vi "02 Valve Test.vi"() -> ()   [LabVIEW 2012]
uses:
  Agilent Channel Definition.ctl
  Drivers/Agilent 34970/Agilent 34970.lvlib
panel:
  in  "Start Button 1-12":bool[](array[boolean])
  out "Max Valves":bool
  out "Agilent Array":refnum<visa-resource-name>[](array[refnum])
  out "Chan Array":string[](array[string])
  in  "Current Per Valve":dbl=0.42
  in  "Current Limit":dbl=1.0
  out "Channel":string
  in  "Walk Time":u32=20000
  out "Agilent Used":string
  in  "TEST TYPE":bool
  in  "Cycles":i32=10
  in  "OK":bool
  in  "One Shot Time":dbl=2000.0
  in  "Valves 41-50":bool[](array[boolean])
  in  "Valves 51-56":bool[](array[boolean])
  in  "Valves 31-40":bool[](array[boolean])
  in  "Valves 21-30":bool[](array[boolean])
  in  "Valves 11-20":bool[](array[boolean])
  in  "Vavles 1-10":bool[](array[boolean])
  out "error out":errorcluster
  in  "error in (no error)":errorcluster
  out "Station In":string
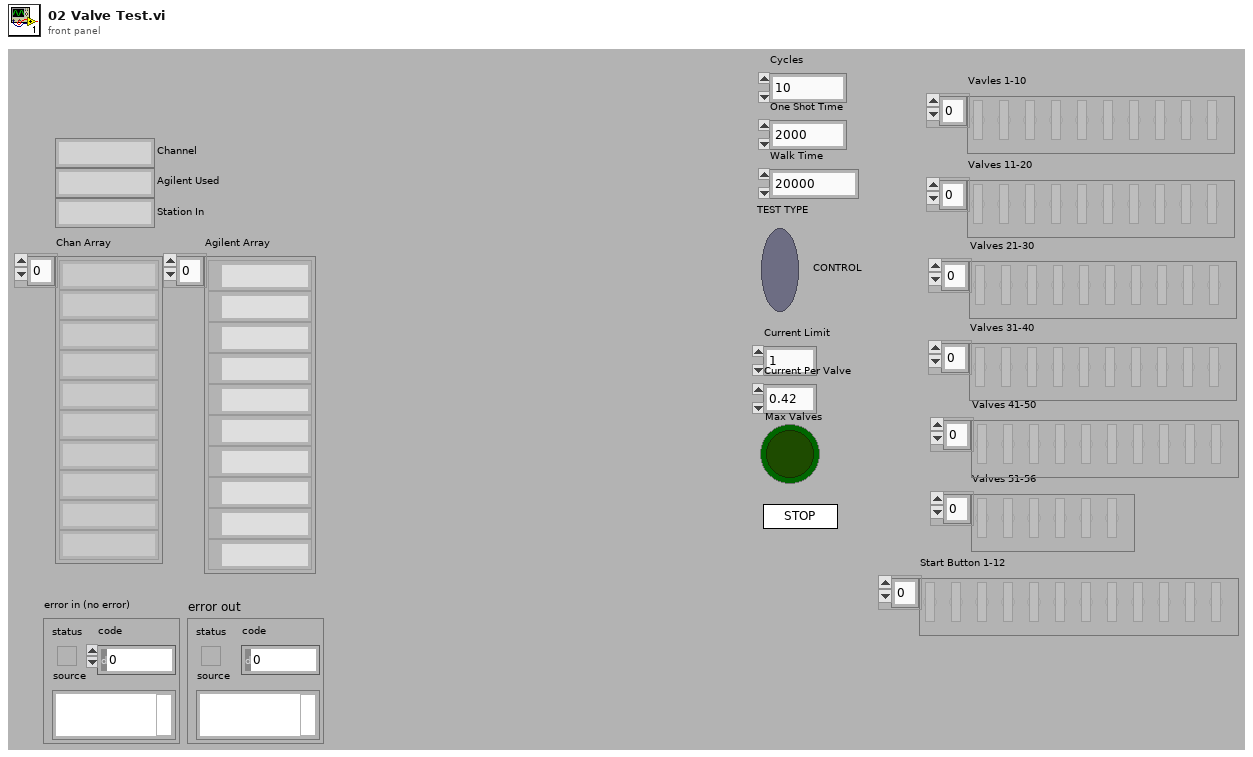
[diagram p1: front panel]
types:
  T1 = typedef "Agilent Channel Definition.ctl" = cluster{"Channel":string, "Station":string, "Label":string, "Agilent Station":string}
  T2 = enum32{"invalid app kind", "Development System", "Run Time System", "Student Edition", "Embedded LabVIEW", "Evaluation", "Custom"}
  T3 = enum32{"Invalid", "Standard", "Closed", "Hidden", "Minimized", "Maximized"}
  T4 = cluster{"Core":cluster{"Current VI Reference":refnum<vi>, "Close Panel on Exit?":bool}, "Valve Array":bool[], "Agilent":refnum<visa-resource-name>, "Channel":string}
  T5 = cluster{"Current VI Reference":refnum<vi>, "Close Panel on Exit?":bool}
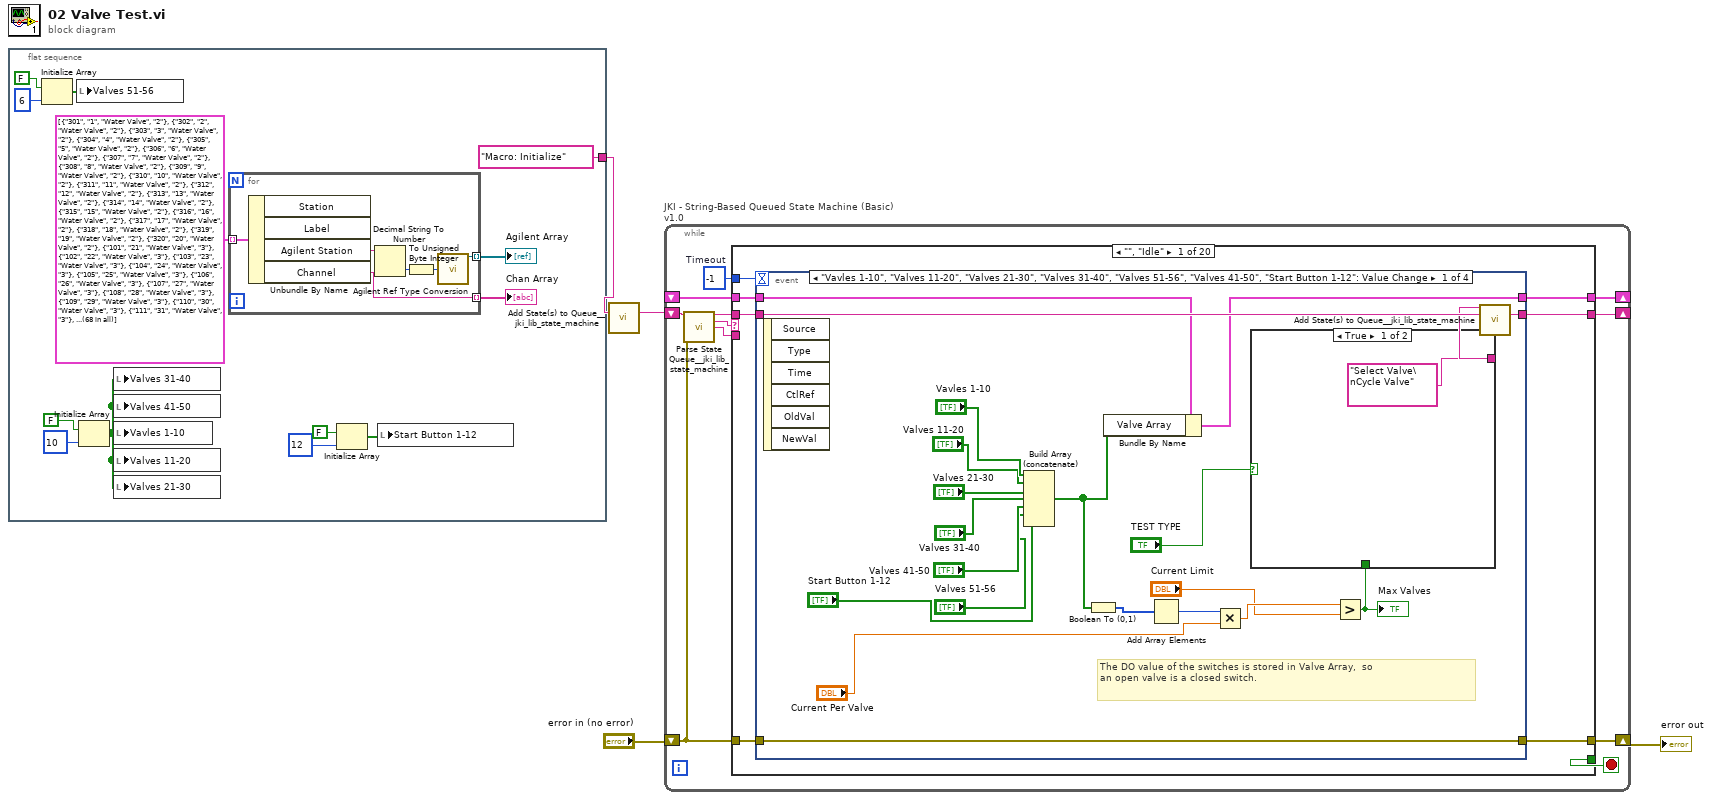
[diagram p0: block diagram]
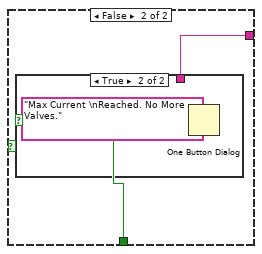
[diagram p2: hidden frame]
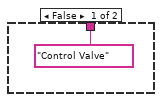
[diagram p3: hidden frame]
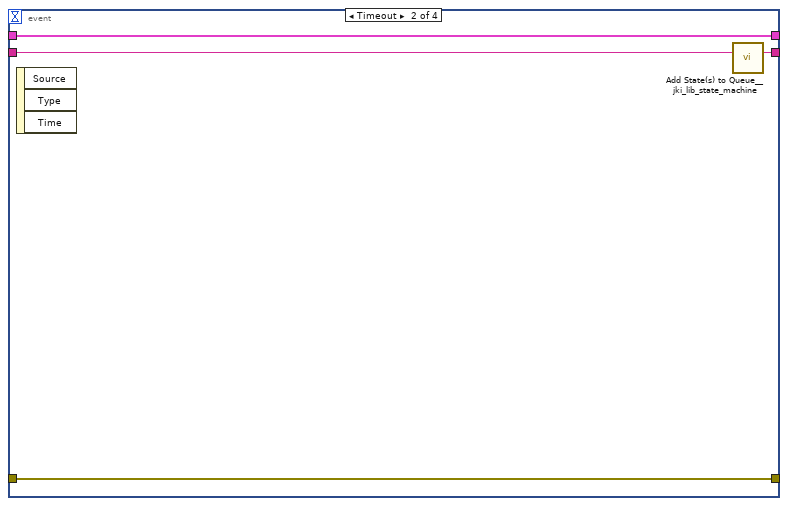
[diagram p4: hidden frame]
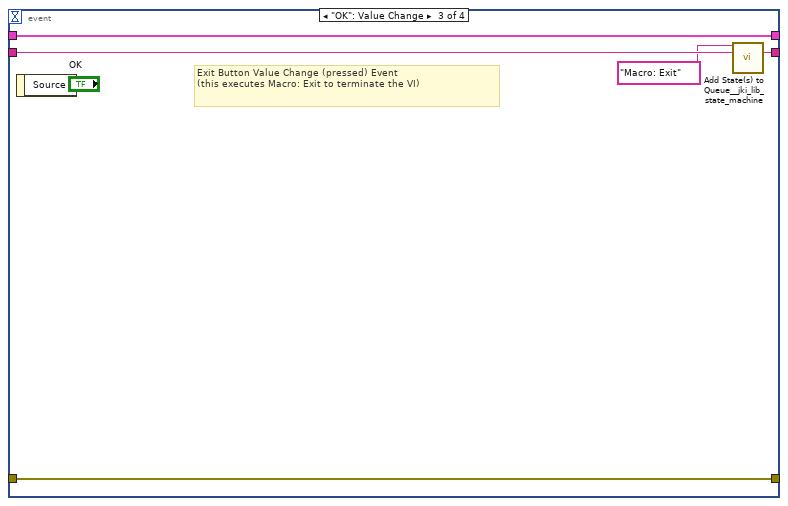
[diagram p5: hidden frame]
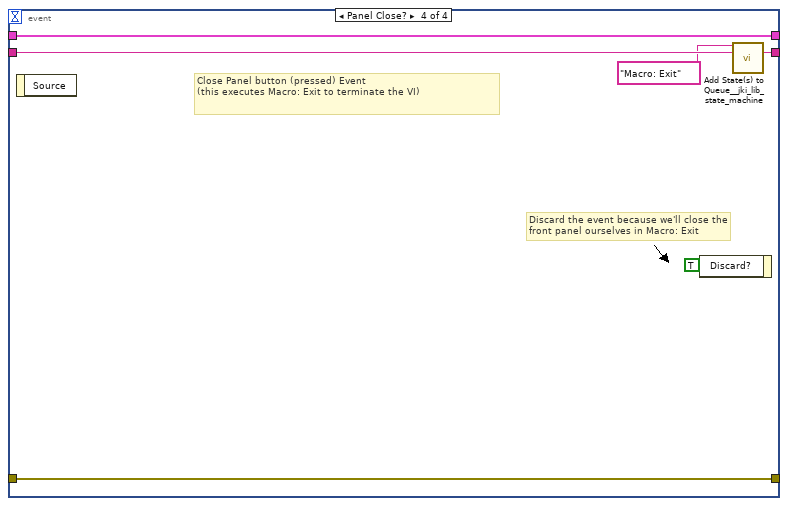
[diagram p6: hidden frame]
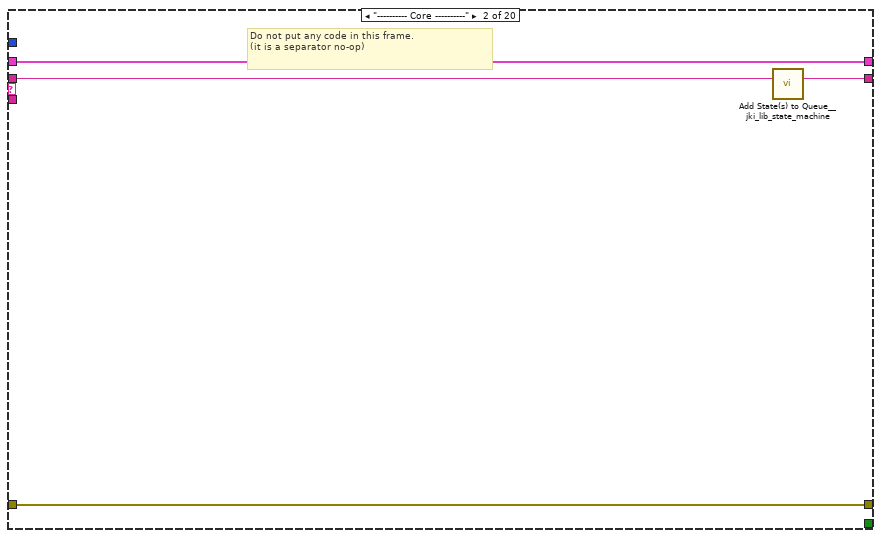
[diagram p7: hidden frame]
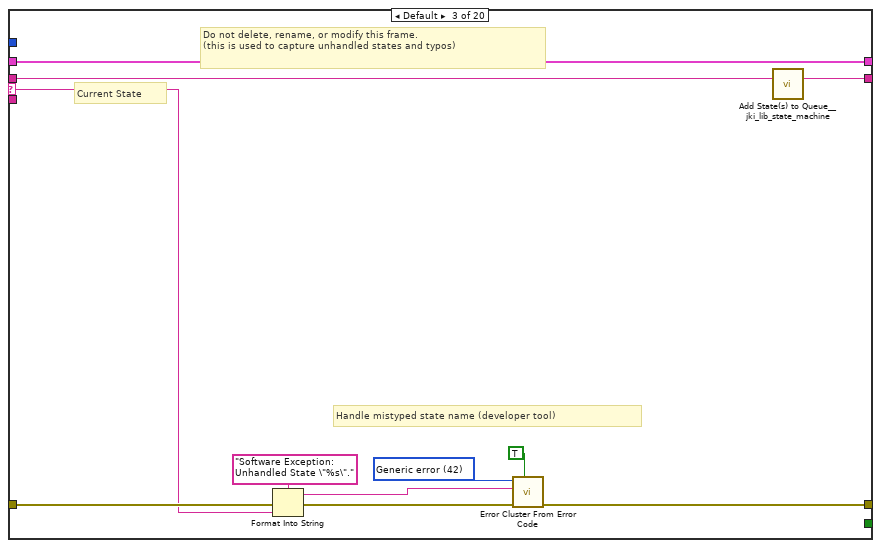
[diagram p8: hidden frame]
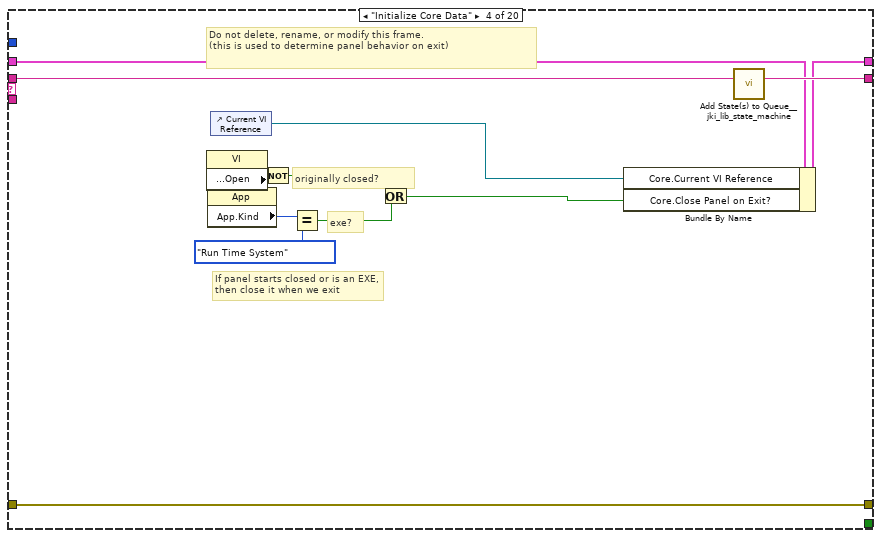
[diagram p9: hidden frame]
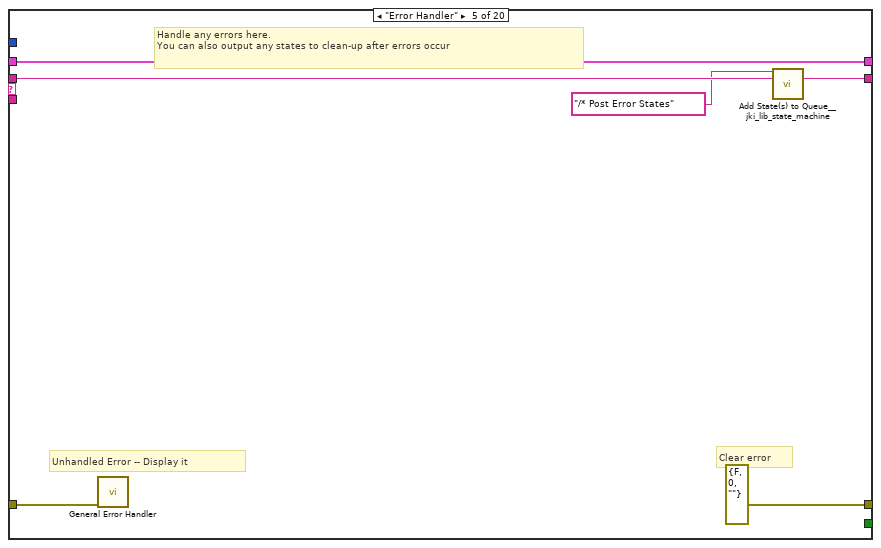
[diagram p10: hidden frame]
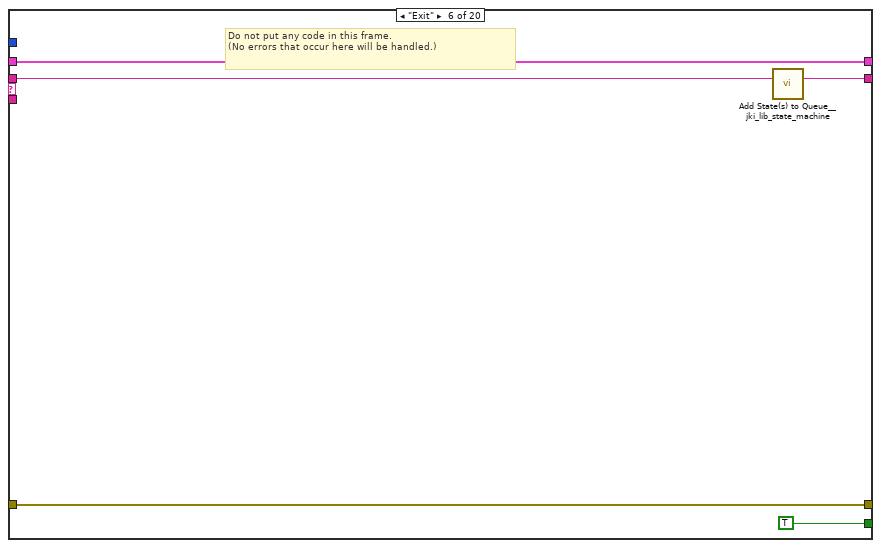
[diagram p11: hidden frame]
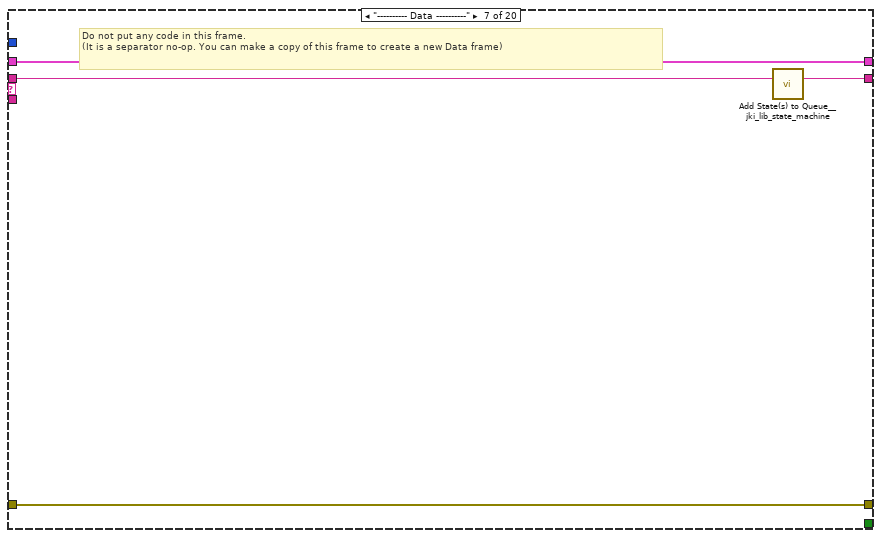
[diagram p12: hidden frame]
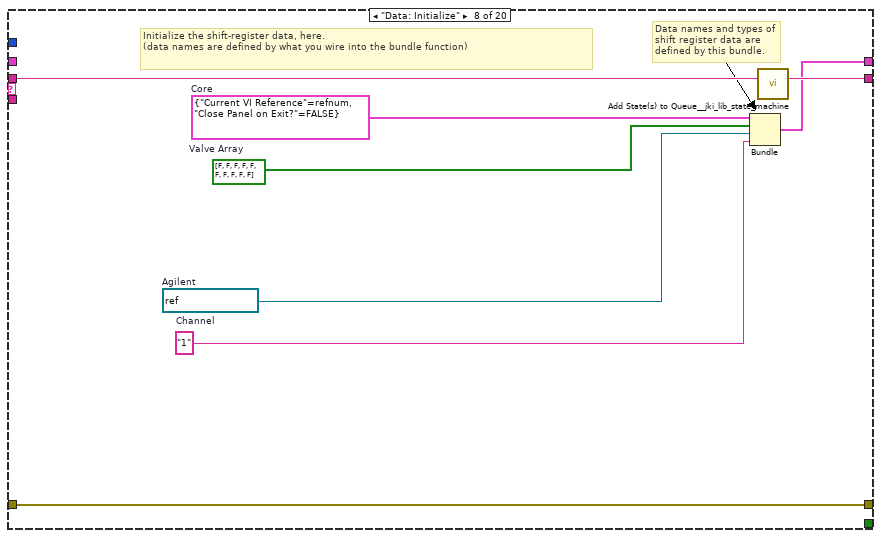
[diagram p13: hidden frame]
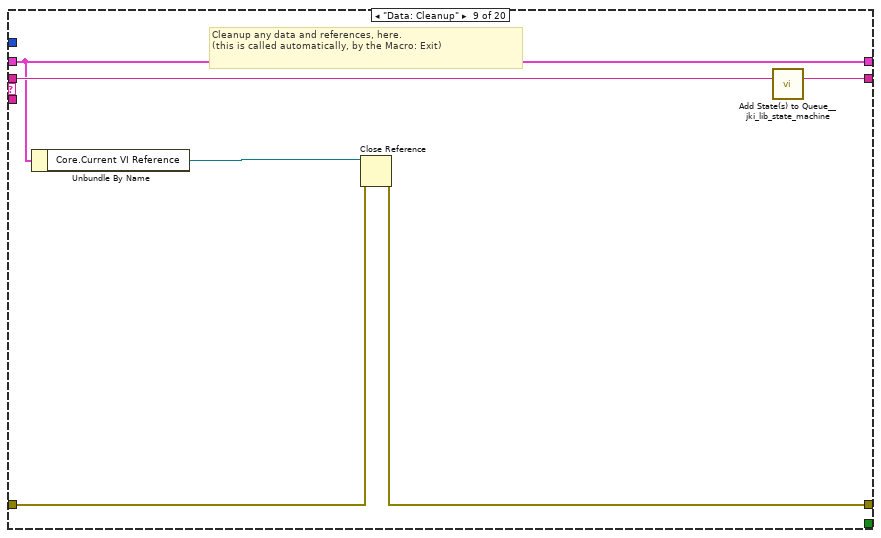
[diagram p14: hidden frame]
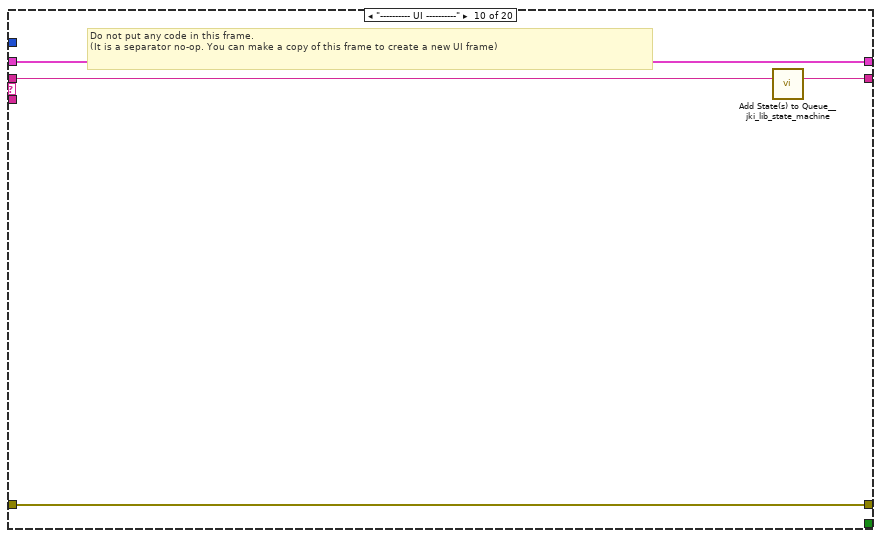
[diagram p15: hidden frame]
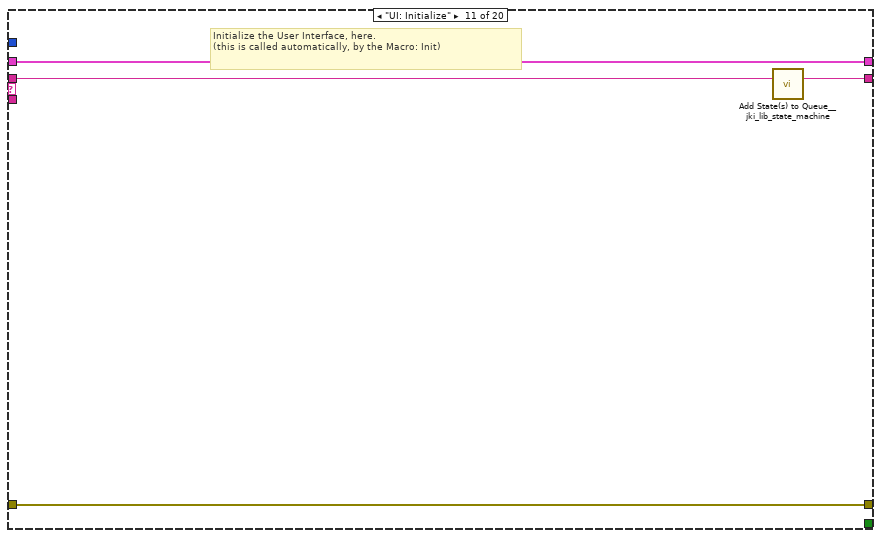
[diagram p16: hidden frame]
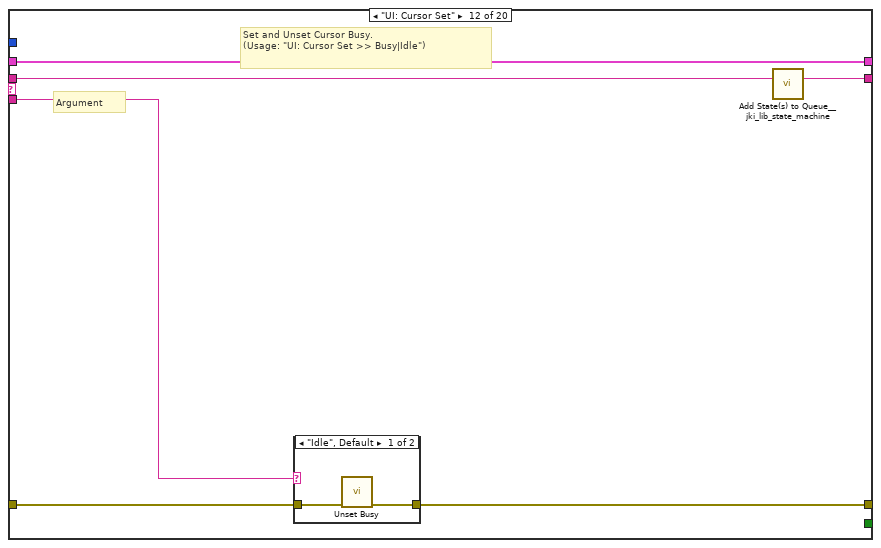
[diagram p17: hidden frame]
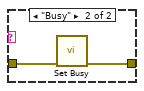
[diagram p18: hidden frame]
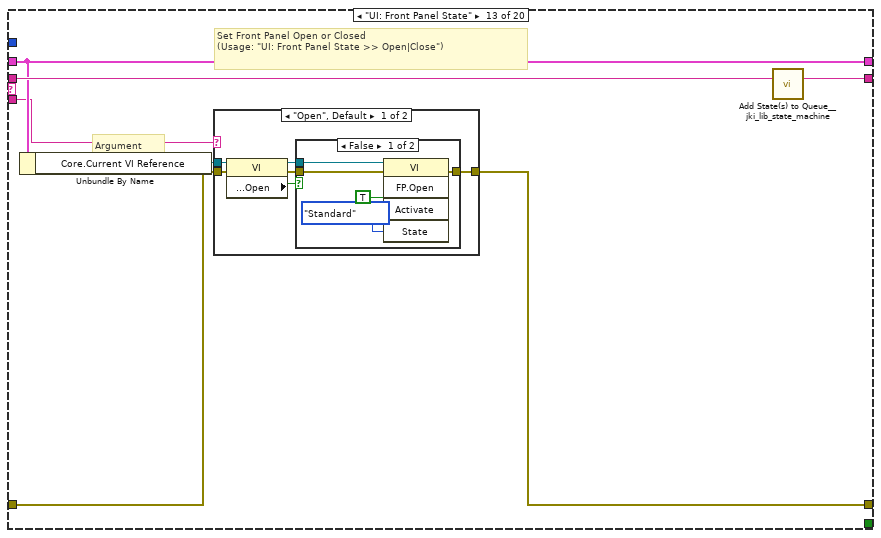
[diagram p19: hidden frame]
diagram:
  n1 = flat-sequence {
    tunnel: ["Macro: Initialize"] -> w1
    frame #0 {
      n2 = Initialize Array(FALSE ("Set/Check (F:Set)"), 6 ("dimension size")) -> (w12:bool[])
      n3 = local write "Valves 51-56"(w12) -> ()
      n4 = Initialize Array(FALSE ("Set/Check (F:Set)"), 10 ("dimension size")) -> (w15:bool[])
      n5 = local write "Valves 31-40"(w15) -> ()
      n6 = local write "Valves 41-50"(w15) -> ()
      n7 = local write "Vavles 1-10"(w15) -> ()
      n8 = local write "Valves 11-20"(w15) -> ()
      n9 = local write "Valves 21-30"(w15) -> ()
      n10 = for {
        tunnel: T1[] [{"Channel"="301", "Station"="1", "Label"="Water Valve", "Agilent Station"="2"}, {"Channel"="302", "Station"="2", "Label"="Water Valve", "Agilent Station"="2"}, {"Channel"="303", "Station"="3", "Label"="Water Valve", "Agilent Station"="2"}, {"Channel"="304", "Station"="4", "Label"="Water Valve", "Agilent Station"="2"}, {"Channel"="305", "Station"="5", "Label"="Water Valve", "Agilent Station"="2"}, {"Channel"="306", "Station"="6", "Label"="Water Valve", "Agilent Station"="2"}, {"Channel"="307", "Station"="7", "Label"="Water Valve", "Agilent Station"="2"}, {"Channel"="308", "Station"="8", "Label"="Water Valve", "Agilent Station"="2"}, {"Channel"="309", "Station"="9", "Label"="Water Valve", "Agilent Station"="2"}, {"Channel"="310", "Station"="10", "Label"="Water Valve", "Agilent Station"="2"}, {"Channel"="311", "Station"="11", "Label"="Water Valve", "Agilent Station"="2"}, {"Channel"="312", "Station"="12", "Label"="Water Valve", "Agilent Station"="2"}, {"Channel"="313", "Station"="13", "Label"="Water Valve", "Agilent Station"="2"}, {"Channel"="314", "Station"="14", "Label"="Water Valve", "Agilent Station"="2"}, {"Channel"="315", "Station"="15", "Label"="Water Valve", "Agilent Station"="2"}, {"Channel"="316", "Station"="16", "Label"="Water Valve", "Agilent Station"="2"}, {"Channel"="317", "Station"="17", "Label"="Water Valve", "Agilent Station"="2"}, {"Channel"="318", "Station"="18", "Label"="Water Valve", "Agilent Station"="2"}, {"Channel"="319", "Station"="19", "Label"="Water Valve", "Agilent Station"="2"}, {"Channel"="320", "Station"="20", "Label"="Water Valve", "Agilent Station"="2"}, {"Channel"="101", "Station"="21", "Label"="Water Valve", "Agilent Station"="3"}, {"Channel"="102", "Station"="22", "Label"="Water Valve", "Agilent Station"="3"}, {"Channel"="103", "Station"="23", "Label"="Water Valve", "Agilent Station"="3"}, {"Channel"="104", "Station"="24", "Label"="Water Valve", "Agilent Station"="3"}, {"Channel"="105", "Station"="25", "Label"="Water Valve", "Agilent Station"="3"}, {"Channel"="106", "Station"="26", "Label"="Water Valve", "Agilent Station"="3"}, {"Channel"="107", "Station"="27", "Label"="Water Valve", "Agilent Station"="3"}, {"Channel"="108", "Station"="28", "Label"="Water Valve", "Agilent Station"="3"}, {"Channel"="109", "Station"="29", "Label"="Water Valve", "Agilent Station"="3"}, {"Channel"="110", "Station"="30", "Label"="Water Valve", "Agilent Station"="3"}, {"Channel"="111", "Station"="31", "Label"="Water Valve", "Agilent Station"="3"}, {"Channel"="112", "Station"="32", "Label"="Water Valve", "Agilent Station"="3"}, {"Channel"="101", "Station"="33", "Label"="Water Valve", "Agilent Station"="5"}, {"Channel"="102", "Station"="34", "Label"="Water Valve", "Agilent Station"="5"}, {"Channel"="103", "Station"="35", "Label"="Water Valve", "Agilent Station"="5"}, {"Channel"="104", "Station"="36", "Label"="Water Valve", "Agilent Station"="5"}, {"Channel"="105", "Station"="37", "Label"="Water Valve", "Agilent Station"="5"}, {"Channel"="106", "Station"="38", "Label"="Water Valve", "Agilent Station"="5"}, {"Channel"="107", "Station"="39", "Label"="Water Valve", "Agilent Station"="5"}, {"Channel"="108", "Station"="40", "Label"="Water Valve", "Agilent Station"="5"}, {"Channel"="109", "Station"="41", "Label"="Water Valve", "Agilent Station"="5"}, {"Channel"="110", "Station"="42", "Label"="Water Valve", "Agilent Station"="5"}, {"Channel"="111", "Station"="43", "Label"="Water Valve", "Agilent Station"="5"}, {"Channel"="112", "Station"="44", "Label"="Water Valve", "Agilent Station"="5"}, {"Channel"="113", "Station"="45", "Label"="Water Valve", "Agilent Station"="5"}, {"Channel"="114", "Station"="46", "Label"="Water Valve", "Agilent Station"="5"}, {"Channel"="115", "Station"="47", "Label"="Water Valve", "Agilent Station"="5"}, {"Channel"="116", "Station"="48", "Label"="Water Valve", "Agilent Station"="5"}, {"Channel"="117", "Station"="49", "Label"="Water Valve", "Agilent Station"="5"}, {"Channel"="118", "Station"="50", "Label"="Water Valve", "Agilent Station"="5"}, {"Channel"="119", "Station"="51", "Label"="Water Valve", "Agilent Station"="5"}, {"Channel"="120", "Station"="52", "Label"="Water Valve", "Agilent Station"="5"}, {"Channel"="201", "Station"="53", "Label"="Water Valve", "Agilent Station"="5"}, {"Channel"="202", "Station"="54", "Label"="Water Valve", "Agilent Station"="5"}, {"Channel"="203", "Station"="55", "Label"="Water Valve", "Agilent Station"="5"}, {"Channel"="204", "Station"="56", "Label"="Water Valve", "Agilent Station"="5"}, {"Channel"="301", "Station"="21", "Label"="Start Button", "Agilent Station"="5"}, {"Channel"="302", "Station"="22", "Label"="Start Button", "Agilent Station"="5"}, {"Channel"="303", "Station"="23", "Label"="Start Button", "Agilent Station"="5"}, {"Channel"="304", "Station"="24", "Label"="Start Button", "Agilent Station"="5"}, {"Channel"="305", "Station"="25", "Label"="Start Button", "Agilent Station"="5"}, {"Channel"="306", "Station"="26", "Label"="Start Button", "Agilent Station"="5"}, {"Channel"="307", "Station"="27", "Label"="Start Button", "Agilent Station"="5"}, {"Channel"="308", "Station"="28", "Label"="Start Button", "Agilent Station"="5"}, {"Channel"="309", "Station"="29", "Label"="Start Button", "Agilent Station"="5"}, {"Channel"="310", "Station"="30", "Label"="Start Button", "Agilent Station"="5"}, {"Channel"="311", "Station"="31", "Label"="Start Button", "Agilent Station"="5"}, {"Channel"="312", "Station"="32", "Label"="Start Button", "Agilent Station"="5"}] ("Agilent Channels Water Valves") -> [w23] mode=indexing
        tunnel: [w22] -> w10 mode=indexing
        tunnel: [w18] -> w9 mode=indexing
        n11 = Unbundle By Name(w23) -> ("Agilent Station"=w21:string, "Channel"=w22:string)  [unwired: 2 out]
        n12 = Decimal String To Number(string=w21) -> (number=w20:i32)  [unwired: 2 in, 1 out]
        n13 = To Unsigned Byte Integer(number=w20) -> (unsigned 8bit integer=w19:u8)
        n14 = call "Agilent Ref Type Conversion.vi"("Agilent Ref"=w19) -> ("VISA resource name"=w18:refnum<visa-resource-name>)  [unwired: 14 in]
      }
      "Agilent Array" <- w9
      "Chan Array" <- w10
      n15 = Initialize Array(FALSE ("element"), 12 ("dimension size")) -> (w5:bool[])
      n16 = local write "Start Button 1-12"(w5) -> ()
    }
  }
  n17 = call <vilib>:"Add State(s) to Queue__jki_lib_state_machine.vi"("State(s) in (\"\")"=w1) -> ("States Out"=w4:string)  [unwired: 14 in]
  n18 = while "JKI - String-Based Queued State Machine (Basic) v1.0" {
    shift-right: [w27] -> _
    shift-left: _ -> [w26]
    shift-right: [w30] -> w2
    shift-left: "error in (no error)" -> [w24]
    shift-right: [w29] -> _
    shift-left: w4 -> [w31]
    stop <- w28 stop-if-true
    w25 = -1  # Timeout
    n19 = call <vilib>:"Parse State Queue__jki_lib_state_machine.vi"("State Queue"=w31, "Error In (no error)"=w24) -> ("Remaining States"=w33:string, "Current State"=w34:string, "Arguments"=w32:string)  [unwired: 11 in]
    n20 = case shown="\"\", \"Idle\"" w34 {
      selector: w34 -> [_ _ w87 _ _ _ _ _ _ _ _ _ _ _ _ _ _ _ _ _]
      tunnel: w33 -> [w41 w86 w91 w109 w115 w120 w124 w132 w138 w142 w146 w152 w163 w189 w194 w204 w208 w222 w255 w284]
      tunnel: w32 -> [_ _ _ _ _ _ _ _ _ _ _ w147 w157 _ _ _ _ _ _ _]
      tunnel: w26 -> [w39 w83 w89 w100 w112 w118 w121 _ w133 w139 w144 w150 w159 w186 w191 w201 w205 w214 w253 w282]
      tunnel: [w38 w84 w93 w106 errorcluster {"status"=FALSE, "code"=0, "source"=""} ("error out") w117 w122 w129 w134 w140 w143 w148 w160 w187 w192 w202 w206 w220 w245 w280] -> w30
      tunnel: w24 -> [w37 w84 w92 w106 w111 w117 w122 w129 w135 w140 w143 w149 w161 w187 w192 w202 w206 w220 w243 w281]
      tunnel: [w40 w85 w90 w108 w114 w119 w123 w131 w137 w141 w145 w151 w162 w188 w193 w203 w207 w221 w254 w283] -> w29
      tunnel: [_ _ _ _ _ TRUE _ _ _ _ _ _ _ _ _ _ _ _ _ _] -> w28
      tunnel: [w36 w83 w89 w107 w112 w118 w121 w130 w133 w139 w144 w150 w159 w186 w191 w201 w205 w213 w253 w282] -> w27
      tunnel: w25 -> [w35 _ _ _ _ _ _ _ _ _ _ _ _ _ _ _ _ _ _ _]
      frame "", "Idle" {
        n21 = event shown="[0] \"Vavles 1-10\", \"Valves 11-20\", \"Valves 21-30\", \"Valves 31-40\", \"Valves 51-56\", \"Valves 41-50\", \"Start Button 1-12\": Value Change" {
          selector: _ -> [_ _ _ _]
          dyn-events: _ -> [_ _ _ _]
          timeout: w35 -> [_ _ _ _]
          tunnel: w41 -> [w62 w71 w76 w82]
          tunnel: [w61 w70 w75 w81] -> w40
          tunnel: w39 -> [w58 w68 w73 w79]
          tunnel: [w60 w69 w74 w80] -> w38
          tunnel: w37 -> [w60 w69 w74 w80]
          tunnel: [w57 w68 w73 w79] -> w36
          event "Vavles 1-10", "Valves 11-20", "Valves 21-30", "Valves 31-40", "Valves 51-56", "Valves 41-50", "Start Button 1-12": Value Change {
            # "The DO value of the switches is stored in Valve Array,  so\nan open valve is a closed switch."
            n22 = event-data() -> ()  [unwired: 1 in, 6 out]
            n23 = Build Array (concatenate)("Vavles 1-10", "Valves 11-20", "Valves 21-30", "Valves 31-40", "Valves 41-50", "Valves 51-56", "Start Button 1-12") -> (w49:bool[])
            n24 = Boolean To (0,1)(Boolean=w49) -> (0, 1=w48:i16[])
            n25 = Bundle By Name(cluster=w58, "Valve Array"=w49) -> (w57:T4)
            n26 = Add Array Elements(numeric array=w48) -> (sum=w43:i16)
            n27 = Multiply(x=w43, y="Current Per Valve") -> (x*y=w46:dbl)
            n28 = Greater?(x=w46, y="Current Limit") -> (0:w44:bool)
            "Max Valves" <- w44
            n29 = case shown="True" "TEST TYPE" {
              tunnel: ["Select Valve\nCycle Valve" ("State(s) in Front (\"\")") w65] -> w59
              tunnel: w44 -> [_ w64]
              frame True {
              }
              frame False {
                n30 = case shown="True" w64 {
                  tunnel: ["Control Valve" ("State(s) in Front (\"\")") _] -> w65
                  frame False {
                  }
                  frame True {
                    n31 = One Button Dialog(message="Max Current \nReached. No More Valves.") -> ()  [unwired: 1 in, 1 out]
                  }
                }
              }
            }
            n32 = call <vilib>:"Add State(s) to Queue__jki_lib_state_machine.vi"("State(s) in Front (\"\")"=w59, "State(s) in (\"\")"=w62) -> ("States Out"=w61:string)  [unwired: 13 in]
          }
          event Timeout {
            n33 = event-data() -> ()  [unwired: 1 in, 3 out]
            n34 = call <vilib>:"Add State(s) to Queue__jki_lib_state_machine.vi"("State(s) in (\"\")"=w71) -> ("States Out"=w70:string)  [unwired: 14 in]
          }
          event "OK": Value Change {
            # "Exit Button Value Change (pressed) Event\n(this executes Macro: Exit to terminate the VI)"
            n35 = event-data() -> ()  [unwired: 1 in, 1 out]
            n36 = call <vilib>:"Add State(s) to Queue__jki_lib_state_machine.vi"("State(s) in Front (\"\")"="Macro: Exit", "State(s) in (\"\")"=w76) -> ("States Out"=w75:string)  [unwired: 13 in]
          }
          event Panel Close? {
            # "Discard the event because we'll close the front panel ourselves in Macro: Exit"
            # "Close Panel button (pressed) Event\n(this executes Macro: Exit to terminate the VI)"
            n37 = event-data() -> ()  [unwired: 1 in, 1 out]
            n38 = event-data("Discard?"=TRUE) -> ()  [unwired: 1 in, 1 out]
            n39 = call <vilib>:"Add State(s) to Queue__jki_lib_state_machine.vi"("State(s) in Front (\"\")"="Macro: Exit", "State(s) in (\"\")"=w82) -> ("States Out"=w81:string)  [unwired: 13 in]
          }
        }
      }
      frame "---------- Core ----------" {
        # "Do not put any code in this frame.\n(it is a separator no-op)"
        n40 = call <vilib>:"Add State(s) to Queue__jki_lib_state_machine.vi"("State(s) in (\"\")"=w86) -> ("States Out"=w85:string)  [unwired: 14 in]
      }
      frame Default {
        w96 = 42 items=["No error", "Argument error", "Memory is full", "Out of zone", "End of file", "File already open", "Generic file I/O error", "File not found", "File permission error", "Disk is full", "Duplicate path", "Too many files open", "System feature not enabled", "Resource file not found", "Cannot add resource", "Resource not found", "Image not found", "Image memory error", "Pen does not exist", "Config type invalid", "Config token not found", "Config parse error", "Config memory error", "Bad external code format", "Bad external code offset", "External code not present", "Null window", "Destroy window error", "Null menu", "Print aborted", "Bad print record", "Print driver error", "Windows error during printing", "Memory error during printing", "Print dialog error", "Generic print error", "Invalid device refnum", "Device not found", "Device parameter error", "Device unit error", "Cannot open device", "Device call aborted", "Generic error", "Cancelled by user", "Object ID too low", "Object ID too high", "Object not in heap", "Unknown heap", "Unknown object (invalid DefProc)", "Unknown object (DefProc not in table)", "Message out of range", "Invalid (null) method", "Unknown message", "Manager call not supported", "Bad address", "Network operation in progress", "Network operation timed out", "Connection is busy", "Network attribute not supported", "Network error", "Address in use", "System out of memory", "Connection aborted", "Connection refused", "Not connected", "Already connected", "Connection closed", "Initialization error (interapplication manager)", "Bad occurrence", "Wait on unbound occurrence handler", "Occurrence queue overflow", "Datalog type conflict", "Unused", "Unrecognized type (interapplication manager)", "Memory corrupt", "Failed to make temporary DLL", "Old CIN version", "Drag socket not found", "Failed to load drop-object", "Failed to register OLE object", "Failed to release OLE object", "Format specifier type mismatch", "Unknown format specifier", "Too few format specifiers", "Too many format specifiers", "Scan failed", "Newer CIN version", "Error converting to variant", "Runtime menu error", "Password tampered", "Variant attribute not found", "Incompatible variant data type", "Event data is not available", "Event Store is not present", "Occurrence is not found", "Event Queue is not created", "Event info is not available", "Refnum passed is NULL", "Error retrieving Class GUID", "Error retrieving CoClass GUID", "Error retrieving TypeLib GUID.", "Bad built application magic bytes.", "Specific driver is different from the specific driver associated with the Logical Name.", "There is no session opened to the class driver.", "Max Error", "MAX - Error with config objects", "MAX - Error loading configuration", "MAX - Group not supported"]
        # "Current State"
        # "Do not delete, rename, or modify this frame.\n(this is used to capture unhandled states and typos)"
        # "Handle mistyped state name (developer tool)"
        n41 = Format Into String(format string="Software Exception: Unhandled State \"%s\"." ("message"), error in=w92, w87) -> (resulting string=w95:string, error out=w94:errorcluster)  [unwired: 1 in]
        n42 = call <vilib>:"Error Cluster From Error Code.vi"("show call chain? (False)"=TRUE, "error in (no error)"=w94, "error message (\"\")"=w95, "error code (0)"=w96) -> ("error out"=w93:errorcluster)  [unwired: 5 in]
        n43 = call <vilib>:"Add State(s) to Queue__jki_lib_state_machine.vi"("State(s) in (\"\")"=w91) -> ("States Out"=w90:string)  [unwired: 14 in]
      }
      frame "Initialize Core Data" {
        # "Do not delete, rename, or modify this frame.\n(this is used to determine panel behavior on exit)"
        # "originally closed?"
        # "exe?"
        # "If panel starts closed or is an EXE, then close it when we exit"
        n44 = property class="VI"() -> ("Front Panel.Open"=w105:bool)  [unwired: 2 in, 2 out]
        n45 = property class="App"() -> ("App.Kind"=w104:T2)  [unwired: 2 in, 2 out]
        n46 = control-ref of="Current VI Reference"() -> (w98:refnum<vi>)
        n47 = Not(x=w105) -> (.not. x?=w102:bool)
        n48 = Equal?(x=w104, y=T2."Run Time System" ("Application:Kind")) -> (x = y?=w101:bool)
        n49 = Or(x=w102, y=w101) -> (x .or. y?=w99:bool)
        n50 = Bundle By Name(cluster=w100, "Core.Current VI Reference"=w98, "Core.Close Panel on Exit?"=w99) -> (w107:T4)
        n51 = call <vilib>:"Add State(s) to Queue__jki_lib_state_machine.vi"("State(s) in (\"\")"=w109) -> ("States Out"=w108:string)  [unwired: 14 in]
      }
      frame "Error Handler" {
        # "Unhandled Error -- Display it"
        # "Handle any errors here.\nYou can also output any states to clean-up after errors occur"
        # "Clear error"
        n52 = call <vilib>:"General Error Handler.vi"("error in (no error)"=w111) -> ()  [unwired: 10 in, 5 out]
        n53 = call <vilib>:"Add State(s) to Queue__jki_lib_state_machine.vi"("State(s) in Front (\"\")"="/* Post Error States", "State(s) in (\"\")"=w115) -> ("States Out"=w114:string)  [unwired: 13 in]
      }
      frame "Exit" {
        # "Do not put any code in this frame.\n(No errors that occur here will be handled.)"
        n54 = call <vilib>:"Add State(s) to Queue__jki_lib_state_machine.vi"("State(s) in (\"\")"=w120) -> ("States Out"=w119:string)  [unwired: 14 in]
      }
      frame "---------- Data ----------" {
        # "Do not put any code in this frame.\n(It is a separator no-op. You can make a copy of this frame to create a new Data frame)"
        n55 = call <vilib>:"Add State(s) to Queue__jki_lib_state_machine.vi"("State(s) in (\"\")"=w124) -> ("States Out"=w123:string)  [unwired: 14 in]
      }
      frame "Data: Initialize" {
        w125 = "1"  # Channel
        w126 = refnum<visa-resource-name> "AGILENT1"  # Agilent
        w127 = bool[] [FALSE, FALSE, FALSE, FALSE, FALSE, FALSE, FALSE, FALSE, FALSE, FALSE]  # Valve Array
        w128 = T5 {"Current VI Reference"=refnum, "Close Panel on Exit?"=FALSE}  # Core
        # "Data names and types of shift register data are defined by this bundle."
        # "Initialize the shift-register data, here.\n(data names are defined by what you wire into the bundle function)"
        n56 = Bundle("Core"=w128, "Valve Array"=w127, "Agilent"=w126, "Channel"=w125) -> (w130:T4)  [unwired: 1 in]
        n57 = call <vilib>:"Add State(s) to Queue__jki_lib_state_machine.vi"("State(s) in (\"\")"=w132) -> ("States Out"=w131:string)  [unwired: 14 in]
      }
      frame "Data: Cleanup" {
        # "Cleanup any data and references, here.\n(this is called automatically, by the Macro: Exit)"
        n58 = Unbundle By Name(w133) -> ("Core.Current VI Reference"=w136:refnum<vi>)
        n59 = Close Reference(reference=w136, error in (no error)=w135) -> (error out=w134:errorcluster)
        n60 = call <vilib>:"Add State(s) to Queue__jki_lib_state_machine.vi"("State(s) in (\"\")"=w138) -> ("States Out"=w137:string)  [unwired: 14 in]
      }
      frame "---------- UI ----------" {
        # "Do not put any code in this frame.\n(It is a separator no-op. You can make a copy of this frame to create a new UI frame)"
        n61 = call <vilib>:"Add State(s) to Queue__jki_lib_state_machine.vi"("State(s) in (\"\")"=w142) -> ("States Out"=w141:string)  [unwired: 14 in]
      }
      frame "UI: Initialize" {
        # "Initialize the User Interface, here.\n(this is called automatically, by the Macro: Init)"
        n62 = call <vilib>:"Add State(s) to Queue__jki_lib_state_machine.vi"("State(s) in (\"\")"=w146) -> ("States Out"=w145:string)  [unwired: 14 in]
      }
      frame "UI: Cursor Set" {
        # "Argument"
        # "Set and Unset Cursor Busy.\n(Usage: \"UI: Cursor Set >> Busy|Idle\")"
        n63 = case shown="\"Idle\", Default" w147 {
          tunnel: w149 -> [w154 w156]
          tunnel: [w153 w155] -> w148
          frame "Idle", Default {
            n64 = call <vilib>:"Unset Busy.vi"("error in (no error)"=w154) -> ("error out"=w153:errorcluster)  [unwired: 10 in]
          }
          frame "Busy" {
            n65 = call <vilib>:"Set Busy.vi"("error in (no error)"=w156) -> ("error out"=w155:errorcluster)  [unwired: 9 in, 1 out]
          }
        }
        n66 = call <vilib>:"Add State(s) to Queue__jki_lib_state_machine.vi"("State(s) in (\"\")"=w152) -> ("States Out"=w151:string)  [unwired: 14 in]
      }
      frame "UI: Front Panel State" {
        # "Argument"
        # "Set Front Panel Open or Closed\n(Usage: \"UI: Front Panel State >> Open|Close\")"
        n67 = Unbundle By Name(w159) -> ("Core.Current VI Reference"=w158:refnum<vi>)
        n68 = case shown="\"Open\", Default" w157 {
          tunnel: w161 -> [w167 w180]
          tunnel: [w169 w181] -> w160
          tunnel: w158 -> [w168 w178]
          frame "Open", Default {
            n69 = property class="VI"(reference=w168, error in=w167) -> (reference out=w165:refnum<vi>, error out=w166:errorcluster, "Front Panel.Open"=w164:bool)
            n70 = case shown="False" w164 {
              tunnel: [w172 w175] -> w169
              tunnel: w166 -> [w171 w175]
              tunnel: w165 -> [w170 _]
              frame False {
                n71 = invoke class="VI" method="FP.Open"(reference=w170, error in=w171, "Activate"=TRUE, "State"=T3."Standard") -> (error out=w172:errorcluster)  [unwired: 1 in, 4 out]
              }
              frame True {
              }
            }
          }
          frame "Close" {
            n72 = property class="VI"(reference=w178, error in=w180) -> (reference out=w177:refnum<vi>, error out=w179:errorcluster, "Front Panel.Open"=w176:bool)
            n73 = case shown="True" w176 {
              tunnel: [w182 w185] -> w181
              tunnel: w179 -> [w182 w184]
              tunnel: w177 -> [_ w183]
              frame False {
              }
              frame True {
                n74 = invoke class="VI" method="FP.Close"(reference=w183, error in=w184) -> (error out=w185:errorcluster)  [unwired: 1 in, 2 out]
              }
            }
          }
        }
        n75 = call <vilib>:"Add State(s) to Queue__jki_lib_state_machine.vi"("State(s) in (\"\")"=w163) -> ("States Out"=w162:string)  [unwired: 14 in]
      }
      frame "---------- Macro ----------" {
        # "Do not put any code in this frame.\n(It is a separator no-op. You can make a copy of this frame to create a new Macro frame)"
        n76 = call <vilib>:"Add State(s) to Queue__jki_lib_state_machine.vi"("State(s) in (\"\")"=w189) -> ("States Out"=w188:string)  [unwired: 14 in]
      }
      frame "Macro: Initialize" {
        w190 = "Data: Initialize\nInitialize Core Data\nUI: Initialize\nUI: Front Panel State >> Open\nControl Valve"  # Data: Initialize Initialize Core Data UI: Initialize UI: Front Panel State >> Open Control Valve
        # "Shuts all valves in beginning, so they are in known state."
        # "Initialization Macro\n(This is called once, when the VI starts)"
        n77 = call <vilib>:"Add State(s) to Queue__jki_lib_state_machine.vi"("State(s) in Front (\"\")"=w190, "State(s) in (\"\")"=w194) -> ("States Out"=w193:string)  [unwired: 13 in]
      }
      frame "Macro: Exit" {
        # "Exit Macro\n(This is called once, when the VI exits)"
        n78 = Unbundle By Name(w201) -> ("Core.Close Panel on Exit?"=w200:bool)
        n79 = Select(t="UI: Front Panel State >> Close", s=w200, f="") -> (s? t:f=w197:string)
        n80 = call <vilib>:"Add State(s) to Queue__jki_lib_state_machine.vi"("State(s) in (\"\")"=w197, "State(s) at Back (\"\")"="Data: Cleanup\nExit") -> ("States Out"=w195:string)  [unwired: 13 in]
        n81 = call <vilib>:"Add State(s) to Queue__jki_lib_state_machine.vi"("State(s) in Front (\"\")"=w195, "State(s) in (\"\")"=w204) -> ("States Out"=w203:string)  [unwired: 13 in]
      }
      frame "---------- New Category ----------" {
        # "Template Separator\n(You can make a copy of, or modify, this frame)"
        n82 = call <vilib>:"Add State(s) to Queue__jki_lib_state_machine.vi"("State(s) in (\"\")"=w208) -> ("States Out"=w207:string)  [unwired: 14 in]
      }
      frame "Select Valve" {
        # "Your code here.\n(You can make a copy of, or modify, this frame)"
        n83 = Unbundle By Name(w214) -> ("Valve Array"=w210:bool[])
        n84 = for {
          tunnel: w210 -> [w238] mode=indexing
          tunnel: [w236] -> w219
          i -> [w237]
          stop <- w238 stop-if-true
          n85 = Increment(x=w237) -> (x+1=w236:i32)
        }
        n86 = call "Counter.vi"() -> ()  [unwired: 11 in, 1 out]
        n87 = Number To Decimal String(number=w219) -> (decimal integer string=w218:string)  [unwired: 1 in]
        "Station In" <- w218
        n88 = for {
          tunnel: T1[] [{"Channel"="301", "Station"="1", "Label"="Water Valve", "Agilent Station"="2"}, {"Channel"="302", "Station"="2", "Label"="Water Valve", "Agilent Station"="2"}, {"Channel"="303", "Station"="3", "Label"="Water Valve", "Agilent Station"="2"}, {"Channel"="304", "Station"="4", "Label"="Water Valve", "Agilent Station"="2"}, {"Channel"="305", "Station"="5", "Label"="Water Valve", "Agilent Station"="2"}, {"Channel"="306", "Station"="6", "Label"="Water Valve", "Agilent Station"="2"}, {"Channel"="307", "Station"="7", "Label"="Water Valve", "Agilent Station"="2"}, {"Channel"="308", "Station"="8", "Label"="Water Valve", "Agilent Station"="2"}, {"Channel"="309", "Station"="9", "Label"="Water Valve", "Agilent Station"="2"}, {"Channel"="310", "Station"="10", "Label"="Water Valve", "Agilent Station"="2"}, {"Channel"="311", "Station"="11", "Label"="Water Valve", "Agilent Station"="2"}, {"Channel"="312", "Station"="12", "Label"="Water Valve", "Agilent Station"="2"}, {"Channel"="313", "Station"="13", "Label"="Water Valve", "Agilent Station"="2"}, {"Channel"="314", "Station"="14", "Label"="Water Valve", "Agilent Station"="2"}, {"Channel"="315", "Station"="15", "Label"="Water Valve", "Agilent Station"="2"}, {"Channel"="316", "Station"="16", "Label"="Water Valve", "Agilent Station"="2"}, {"Channel"="317", "Station"="17", "Label"="Water Valve", "Agilent Station"="2"}, {"Channel"="318", "Station"="18", "Label"="Water Valve", "Agilent Station"="2"}, {"Channel"="319", "Station"="19", "Label"="Water Valve", "Agilent Station"="2"}, {"Channel"="320", "Station"="20", "Label"="Water Valve", "Agilent Station"="2"}, {"Channel"="101", "Station"="21", "Label"="Water Valve", "Agilent Station"="3"}, {"Channel"="102", "Station"="22", "Label"="Water Valve", "Agilent Station"="3"}, {"Channel"="103", "Station"="23", "Label"="Water Valve", "Agilent Station"="3"}, {"Channel"="104", "Station"="24", "Label"="Water Valve", "Agilent Station"="3"}, {"Channel"="105", "Station"="25", "Label"="Water Valve", "Agilent Station"="3"}, {"Channel"="106", "Station"="26", "Label"="Water Valve", "Agilent Station"="3"}, {"Channel"="107", "Station"="27", "Label"="Water Valve", "Agilent Station"="3"}, {"Channel"="108", "Station"="28", "Label"="Water Valve", "Agilent Station"="3"}, {"Channel"="109", "Station"="29", "Label"="Water Valve", "Agilent Station"="3"}, {"Channel"="110", "Station"="30", "Label"="Water Valve", "Agilent Station"="3"}, {"Channel"="111", "Station"="31", "Label"="Water Valve", "Agilent Station"="3"}, {"Channel"="112", "Station"="32", "Label"="Water Valve", "Agilent Station"="3"}, {"Channel"="101", "Station"="33", "Label"="Water Valve", "Agilent Station"="5"}, {"Channel"="102", "Station"="34", "Label"="Water Valve", "Agilent Station"="5"}, {"Channel"="103", "Station"="35", "Label"="Water Valve", "Agilent Station"="5"}, {"Channel"="104", "Station"="36", "Label"="Water Valve", "Agilent Station"="5"}, {"Channel"="105", "Station"="37", "Label"="Water Valve", "Agilent Station"="5"}, {"Channel"="106", "Station"="38", "Label"="Water Valve", "Agilent Station"="5"}, {"Channel"="107", "Station"="39", "Label"="Water Valve", "Agilent Station"="5"}, {"Channel"="108", "Station"="40", "Label"="Water Valve", "Agilent Station"="5"}, {"Channel"="109", "Station"="41", "Label"="Water Valve", "Agilent Station"="5"}, {"Channel"="110", "Station"="42", "Label"="Water Valve", "Agilent Station"="5"}, {"Channel"="111", "Station"="43", "Label"="Water Valve", "Agilent Station"="5"}, {"Channel"="112", "Station"="44", "Label"="Water Valve", "Agilent Station"="5"}, {"Channel"="113", "Station"="45", "Label"="Water Valve", "Agilent Station"="5"}, {"Channel"="114", "Station"="46", "Label"="Water Valve", "Agilent Station"="5"}, {"Channel"="115", "Station"="47", "Label"="Water Valve", "Agilent Station"="5"}, {"Channel"="116", "Station"="48", "Label"="Water Valve", "Agilent Station"="5"}, {"Channel"="117", "Station"="49", "Label"="Water Valve", "Agilent Station"="5"}, {"Channel"="118", "Station"="50", "Label"="Water Valve", "Agilent Station"="5"}, {"Channel"="119", "Station"="51", "Label"="Water Valve", "Agilent Station"="5"}, {"Channel"="120", "Station"="52", "Label"="Water Valve", "Agilent Station"="5"}, {"Channel"="201", "Station"="53", "Label"="Water Valve", "Agilent Station"="5"}, {"Channel"="202", "Station"="54", "Label"="Water Valve", "Agilent Station"="5"}, {"Channel"="203", "Station"="55", "Label"="Water Valve", "Agilent Station"="5"}, {"Channel"="204", "Station"="56", "Label"="Water Valve", "Agilent Station"="5"}, {"Channel"="301", "Station"="21", "Label"="Start Button", "Agilent Station"="5"}, {"Channel"="302", "Station"="22", "Label"="Start Button", "Agilent Station"="5"}, {"Channel"="303", "Station"="23", "Label"="Start Button", "Agilent Station"="5"}, {"Channel"="304", "Station"="24", "Label"="Start Button", "Agilent Station"="5"}, {"Channel"="305", "Station"="25", "Label"="Start Button", "Agilent Station"="5"}, {"Channel"="306", "Station"="26", "Label"="Start Button", "Agilent Station"="5"}, {"Channel"="307", "Station"="27", "Label"="Start Button", "Agilent Station"="5"}, {"Channel"="308", "Station"="28", "Label"="Start Button", "Agilent Station"="5"}, {"Channel"="309", "Station"="29", "Label"="Start Button", "Agilent Station"="5"}, {"Channel"="310", "Station"="30", "Label"="Start Button", "Agilent Station"="5"}, {"Channel"="311", "Station"="31", "Label"="Start Button", "Agilent Station"="5"}, {"Channel"="312", "Station"="32", "Label"="Start Button", "Agilent Station"="5"}] ("Agilent Channels Water Valves") -> [w235] mode=indexing
          tunnel: w218 -> [w232]
          tunnel: [w230] -> w215
          tunnel: [w229] -> w211
          stop <- w228 stop-if-true
          n89 = Unbundle By Name(w235) -> ("Station"=w233:string, "Label"=w227:string, "Agilent Station"=w230:string, "Channel"=w229:string)
          n90 = Equal?(x=w232, y=w233) -> (x = y?=w231:bool)
          n91 = Equal?(x=w227, y="Water Valve") -> (x = y?=w224:bool)
          n92 = Equal?(x=w227, y="Start Button") -> (x = y?=w225:bool)
          n93 = Or(x=w224, y=w225) -> (x .or. y?=w223:bool)
          n94 = And(x=w231, y=w223) -> (x .and. y?=w228:bool)
        }
        "Agilent Used" <- w215
        "Channel" <- w211
        n95 = Decimal String To Number(string=w215) -> (number=w216:i32)  [unwired: 2 in, 1 out]
        n96 = To Unsigned Byte Integer(number=w216) -> (unsigned 8bit integer=w217:u8)
        n97 = call "Agilent Ref Type Conversion.vi"("Agilent Ref"=w217) -> ("VISA resource name"=w212:refnum<visa-resource-name>)  [unwired: 14 in]
        n98 = Bundle By Name(cluster=w214, "Agilent"=w212, "Channel"=w211) -> (w213:T4)
        n99 = call <vilib>:"Add State(s) to Queue__jki_lib_state_machine.vi"("State(s) in (\"\")"=w222) -> ("States Out"=w221:string)  [unwired: 14 in]
      }
      frame "Cycle Valve" {
        # "Your code here.\n(You can make a copy of, or modify, this frame)"
        n100 = Unbundle By Name(w253) -> ("Agilent"=w252:refnum<visa-resource-name>, "Channel"=w244:string)
        n101 = call "Delay mS.vi"("Error In"=w243, "milliseconds to wait"="Walk Time") -> ("Error Out"=w242:errorcluster)  [unwired: 13 in]
        n102 = disable-structure shown="Enabled" {
          disable-tunnel: w252 -> [w261 _]
          disable-tunnel: FALSE ("Set/Check (F:Set)") -> [w260 _]
          disable-tunnel: "Cycles" -> [w259 _]
          disable-tunnel: [w258 w273] -> w245
          disable-tunnel: w244 -> [w257 _]
          disable-tunnel: w242 -> [w256 w273]
          frame Enabled {
            n103 = for {
              N: w259 -> [_]
              tunnel: w261 -> [w269]
              tunnel: w260 -> [w268]
              shift-right: [w263] -> w258
              shift-left: w256 -> [w266]
              tunnel: w257 -> [w265]
              n104 = call "Switch.vi"("Channel List(empty)"=w265, "error in (no error)"=w266, "Open/Close (F:Close)"=w268, "VISA Resource Name"=w269) -> ("error out"=w271:errorcluster, "VISA Resource Name Out"=w270:refnum<visa-resource-name>)  [unwired: 5 in, 1 out]
              n105 = Not(x=w268) -> (.not. x?=w272:bool)
              n106 = call "Delay mS.vi"("Error In"=w271, "milliseconds to wait"="One Shot Time") -> ("Error Out"=w267:errorcluster)  [unwired: 13 in]
              n107 = call "Switch.vi"("Channel List(empty)"=w265, "error in (no error)"=w267, "Open/Close (F:Close)"=w272, "VISA Resource Name"=w270) -> ("error out"=w264:errorcluster)  [unwired: 5 in, 2 out]
              n108 = call "Delay mS.vi"("Error In"=w264, "milliseconds to wait"="One Shot Time") -> ("Error Out"=w263:errorcluster)  [unwired: 13 in]
            }
          }
          frame Disabled {
          }
        }
        n109 = local read "Vavles 1-10"() -> (w239:bool[])
        n110 = local read "Valves 51-56"() -> (w248:bool[])
        n111 = Not(x=w239) -> (.not. x?=w240:bool[])
        n112 = Not(x=w248) -> (.not. x?=w249:bool[])
        n113 = Equal?(x=w239, y=w240) -> (x = y?=w247:bool[])
        n114 = Equal?(x=w248, y=w249) -> (x = y?=w246:bool[])
        n115 = flat-sequence {
          tunnel: w247 -> [w275]
          tunnel: w246 -> [w274]
          tunnel: w245 -> [_]
          frame #0 {
            n116 = local write "Valves 21-30"(w275) -> ()
            n117 = local write "Valves 11-20"(w275) -> ()
            n118 = local write "Valves 51-56"(w274) -> ()
            n119 = local write "Valves 31-40"(w275) -> ()
            n120 = local write "Valves 41-50"(w275) -> ()
            n121 = local write "Vavles 1-10"(w275) -> ()
          }
        }
        n122 = call <vilib>:"Add State(s) to Queue__jki_lib_state_machine.vi"("State(s) in (\"\")"=w255) -> ("States Out"=w254:string)  [unwired: 14 in]
      }
      frame "Control Valve" {
        # "Your code here.\n(You can make a copy of, or modify, this frame)"
        n123 = local read "Chan Array"() -> (w278:string[])
        n124 = local read "Agilent Array"() -> (w279:refnum<visa-resource-name>[])
        n125 = Unbundle By Name(w282) -> ("Valve Array"=w277:bool[])
        n126 = Not(x=w277) -> (.not. x?=w276:bool[])
        n127 = for {
          tunnel: w279 -> [w289] mode=indexing
          tunnel: w276 -> [w288] mode=indexing
          shift-right: [w285] -> w280
          shift-left: w281 -> [w287]
          tunnel: w278 -> [w286] mode=indexing
          n128 = call "Switch.vi"("Channel List(empty)"=w286, "error in (no error)"=w287, "Open/Close (F:Close)"=w288, "VISA Resource Name"=w289) -> ("error out"=w285:errorcluster)  [unwired: 5 in, 2 out]
        }
        n129 = call <vilib>:"Add State(s) to Queue__jki_lib_state_machine.vi"("State(s) in (\"\")"=w284) -> ("States Out"=w283:string)  [unwired: 14 in]
      }
    }
  }
  "error out" <- w2
